vi "pop.vi"(8 "error in (no error)":errorcluster, 11 "Appliance in":refnum<class "Appliance.lvclass">) -> (0 "error out":errorcluster, 3 "Appliance out":refnum<class "Appliance.lvclass">)   [LabVIEW 2010, in "Appliance.lvclass"]
uses:
  Appliance.lvclass
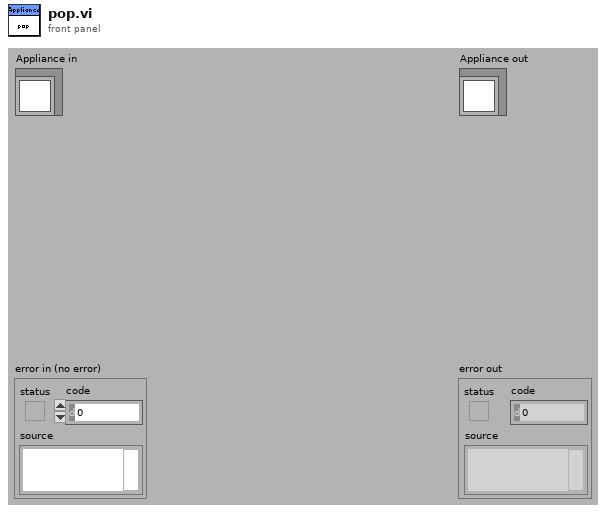
[diagram p1: front panel]
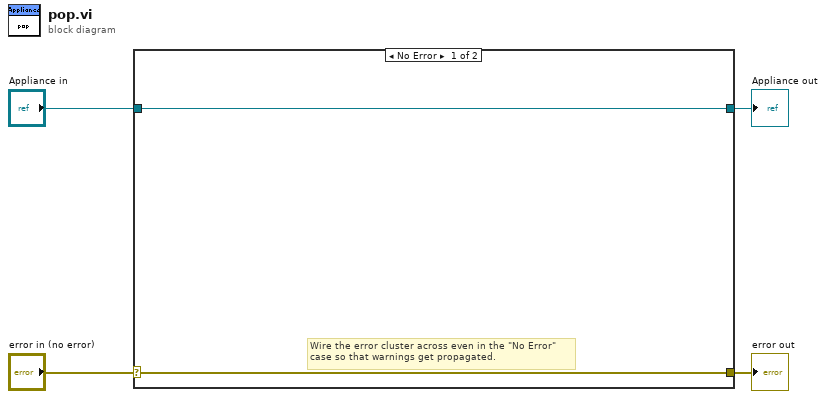
[diagram p0: block diagram]
diagram:
  n1 = case shown="No Error" "error in (no error)" {
    selector: "error in (no error)" -> [w5 w8]
    tunnel: [w5 w8] -> w3
    tunnel: [w6 w7] -> w1
    tunnel: "Appliance in" -> [w6 w7]
    frame No Error {
      # "Wire the error cluster across even in the \"No Error\"\ncase so that warnings get propagated."
    }
    frame Error {
    }
  }
  "error out" <- w3
  "Appliance out" <- w1
